vi "SrBuildReplaceString.vi"(5 "ReplStrLengths":i32[](array[numeric]), 6 "ReplSubStrNum":i32[](array[numeric]), 7 "ReplStrOffsets":i32[](array[numeric]), 8 "OffsetsPastMatch":i32[](array[numeric]), 9 "MatchOffsets":i32[](array[numeric]), 10 "Subject":string, 11 "ReplaceString":string) -> (3 "ReplaceString":string)   [LabVIEW 2021, in "libpcre2-8.lvlib"]
uses:
  libpcre2-8.lvlib
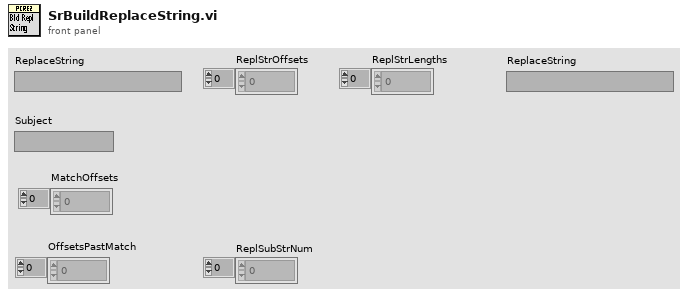
[diagram p1: front panel]
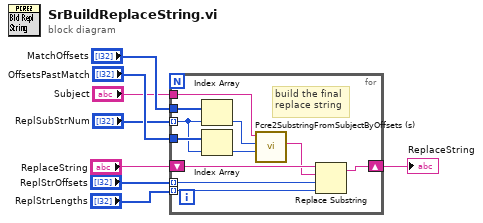
[diagram p0: block diagram]
diagram:
  n1 = for {
    tunnel: "ReplStrOffsets" -> [w18] mode=indexing
    tunnel: "ReplStrLengths" -> [w17] mode=indexing
    shift-right: [w16] -> w7
    shift-left: "ReplaceString" -> [w19]
    tunnel: "MatchOffsets" -> [w15]
    tunnel: "OffsetsPastMatch" -> [w14]
    tunnel: "ReplSubStrNum" -> [w13] mode=indexing
    tunnel: "Subject" -> [w10]
    # "build the final\nreplace string"
    n2 = Index Array(array=w15, index=w13) -> (element=w12:i32)
    n3 = Index Array(array=w14, index=w13) -> (element=w11:i32)
    n4 = call "Pcre2SubstringFromSubjectByOffsets (s).vi"("OffsetPastMatch"=w11, "MatchOffset"=w12, "Subject"=w10) -> ("Substring"=w9:string)  [unwired: 8 in]
    n5 = Replace Substring(2:w17, 3:w18, 4:w9, 5:w19) -> (1:w16:string)  [unwired: 1 out]
  }
  "ReplaceString" <- w7
